vi "ExSetup1strip.vi"() -> ()   [LabVIEW 2010]
uses:
  Open-Close Hardware/CamHandle.vi
panel:
  out "ADC Speed":u32
  out "error out":errorcluster
  in  "error in (no error)":errorcluster
  in  "Timing Mode":u32(ring)=1 items=["N/A", "Timed Mode/Free run", "Trigger First (only PM)", "Strobed/Ext Sync", "Bulb Mode (PM only)", "Variable Timed mode (PM only)", "Flash Mode (only some PM)"]
  in  "x1":u32=1
  in  "x2":u32=1340
  in  "y1":u32=50
  in  "y2":u32=50
  in  "min block":u32=2
  in  "Num Min Block":u32=5
  # "ExSetup1strip.vi : This vi setups up one strip. the x binning is set to 1. and the y binning is y2 - y1 + 1 (i.e. all active strips binned into 1 strip)."
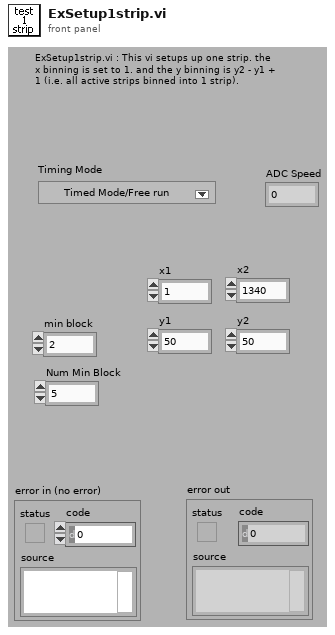
[diagram p1: front panel]
types:
  T1 = cluster{"x1":u32, "x2":u32, "x bin":i32, "y1":u32, "y2":u32, u32}
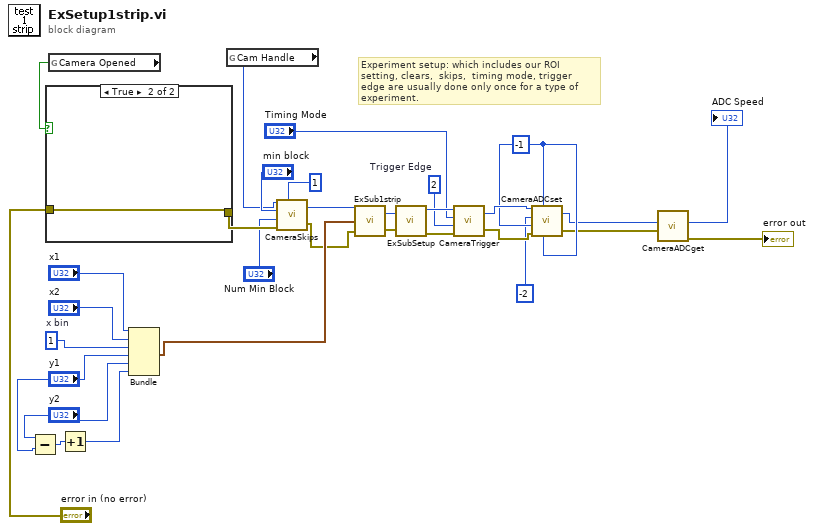
[diagram p0: block diagram]
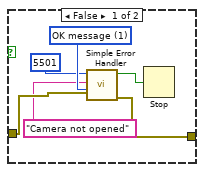
[diagram p2: hidden frame]
diagram:
  w4 = 1  # x bin
  w25 = -1
  w29 = u32 2  # Trigger Edge
  # "Experiment setup: which includes our ROI setting, clears,  skips,  timing mode, trigger edge are usually done only once for a type of experiment."
  n1 = Subtract(x="y2", y="y1") -> (x-y=w3:u32)
  n2 = global read "CamHandle.vi" "Camera Opened"() -> (w28:bool)
  n3 = case shown="True" w28 {
    tunnel: "error in (no error)" -> [w36 w38]
    tunnel: [w35 w38] -> w17
    frame False {
      w37 = u16 1 items=["no dialog", "OK message", "continue or stop message"] ("type of dialog (OK msg:1)")
      n4 = call <vilib>:"Simple Error Handler.vi"("error code (no error:0)"=5501, "error source (\" \")"="Camera not opened", "type of dialog (OK msg:1)"=w37, "error in (no error)"=w36) -> ("error?"=w33:bool, "error out"=w35:errorcluster)  [unwired: 1 in, 3 out]
      n5 = Stop(stop? (T)=w33) -> ()
    }
    frame True {
    }
  }
  n6 = Increment(x=w3) -> (x+1=w2:u32)
  n7 = Bundle("x1"="x1", "x2"="x2", "x bin"=w4, "y1"="y1", "y2"="y2", w2) -> (w18:T1)  [unwired: 1 in]
  n8 = global read "CamHandle.vi" "Cam Handle"() -> (w10:u32)
  n9 = call <userlib>:"CameraSkips.vi"("Camera Handle"=w10, "Minimum Block Size"="min block", "Number of Minimum blocks"="Num Min Block", "error in"=w17, "Type of Skips"=1) -> ("Camera Handle"=w15:u32, "error out"=w16:errorcluster)
  n10 = call "ExSub1strip.vi"("error in (no error)"=w16, "strip 1"=w18, "Camera Handle"=w15) -> ("error out"=w23:errorcluster, "Camera Handle"=w11:u32)
  n11 = call "ExSubSetup.vi"("error in (no error)"=w23, "Camera Handle"=w11) -> ("error out"=w30:errorcluster, "Camera Handle"=w31:u32)
  n12 = call <userlib>:"CameraTrigger.vi"("error in"=w30, "Trigger Edge"=w29, "Timing Mode"="Timing Mode", "Camera Handle"=w31) -> ("error out"=w27:errorcluster, "Camera Handle"=w26:u32)
  n13 = call <userlib>:"CameraADCset.vi"("ADC offset"=w25, "Read Out port"=w25, "error in (no error)"=w27, "ADC Gain"=w25, "ADC Speed"=-2, "Camera Handle"=w26) -> ("error out"=w7:errorcluster, "Camera Handle"=w1:u32)
  n14 = call <userlib>:"CameraADCget.vi"("Camera handle"=w1, "error in (no error)"=w7) -> ("ADC Speed"=→"ADC Speed":i32, "error out"=→"error out":errorcluster)  [unwired: 6 out]
